vi "Milling parameter to trapezoidal shape.vi"(6 "Y location (um)":dbl, 8 "Image height":u32=512, 9 "Image width":u32=512, 11 "Milling para":T1={"X resolution"=4096, "Y resolution"=125001, "X offset (um)"=0.0, "Y offset (um)"=0.0, "X center (um)"=0.0, "Y center (um)"=0.0, "X size (um)"=250.0, "Y size (um)"=250.0, "UL-Ang"=90.0, "UR-Ang"=90.0, "Line milling time (s)"=5.0, "Z-step (nm)"=2.0, "Lines auto pause"=1, "Auto pause"=FALSE, "Mill from Bottom"=FALSE, "FIB FOV (um)"=500.0, "Auto Profile"=FALSE, "Mill start from Last"=FALSE, "FIB PID on"=FALSE, "FIB PID reset"=TRUE, "FIB PID measured"=0, "FIB PID target"=0.0, "FIB PID target slope"=0.0, "FIB PID P"=0.001, "FIB PID I"=0.01, "FIB PID D"=0.0, "Emission (uA)"=1.36, "Suppressor (V)"=50.0, "Auto reheat"=FALSE} caption="Milling Parameters" {"Suppressor (V)" step=0.1 format="%.1g"; "Emission (uA)" step=0.1 format="%.2g"; "FIB PID measured" items=["Spec.", "B.D. 1", "B.D. 2", "Mill", "Spec. +"]; "FIB PID target slope" min=-1 max=1 step=0.1; "UR-Ang" format="%.2f"; "UL-Ang" format="%.2f"; "Y offset (um)" step=0.02 format="%.3g"; "X offset (um)" step=1 format="%.3g"; "FIB FOV (um)" format="%.3g"; "Line milling time (s)" format="%.1f"; "Y center (um)" format="%#.3g"; "X center (um)" format="%#.3g"}) -> (0 "X end":dbl, 1 "X start":dbl, 2 "X size (um) @ Y":dbl, 3 "Trapezoidal":cluster{"X":i16, "Y":i16}[](array[cluster]), 4 "Total progress":dbl)   [LabVIEW 2018]
panel:
  # "Direction"
  # "Start\nfrom"
  # "<"
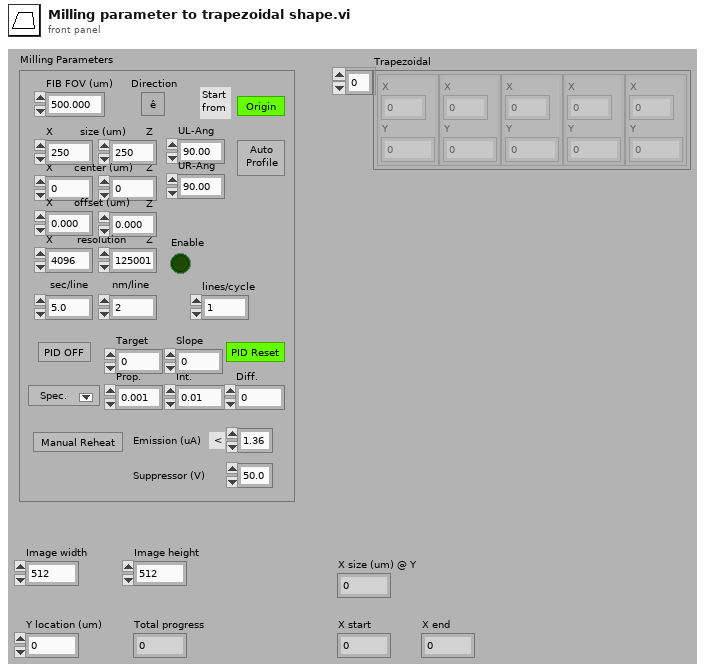
[diagram p1: front panel]
types:
  T1 = cluster{"X resolution":u32, "Y resolution":u32, "X offset (um)":sgl, "Y offset (um)":sgl, "X center (um)":sgl, "Y center (um)":sgl, "X size (um)":sgl, "Y size (um)":sgl, "UL-Ang":sgl, "UR-Ang":sgl, "Line milling time (s)":sgl, "Z-step (nm)":dbl, "Lines auto pause":u16, "Auto pause":bool, "Mill from Bottom":bool, "FIB FOV (um)":sgl, "Auto Profile":bool, "Mill start from Last":bool, "FIB PID on":bool, "FIB PID reset":bool, "FIB PID measured":u8, "FIB PID target":sgl, "FIB PID target slope":sgl, "FIB PID P":sgl, "FIB PID I":sgl, "FIB PID D":sgl, "Emission (uA)":dbl, "Suppressor (V)":sgl, "Auto reheat":bool}
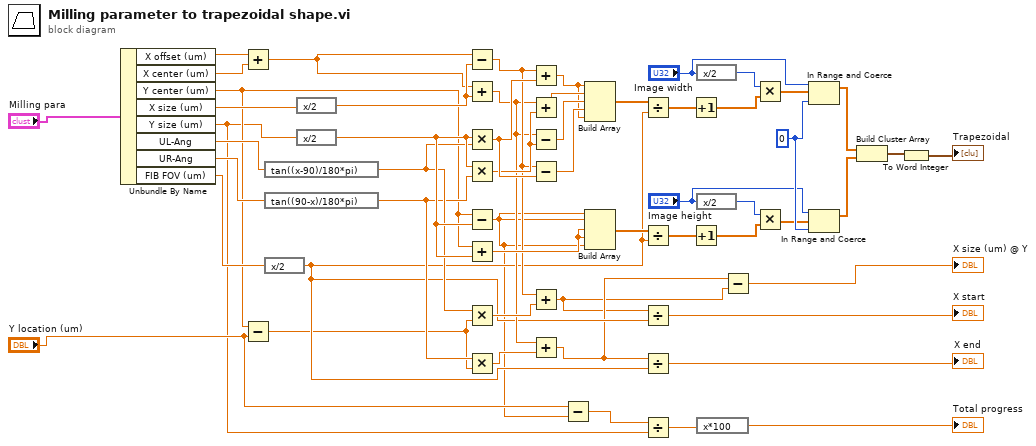
[diagram p0: block diagram]
diagram:
  w33 = u32 0 ("Image width")
  n1 = Unbundle By Name("Milling para") -> ("X offset (um)"=w10:sgl, "X center (um)"=w9:sgl, "Y center (um)"=w11:sgl, "X size (um)"=w54:sgl, "Y size (um)"=w4:sgl, "UL-Ang"=w53:sgl, "UR-Ang"=w52:sgl, "FIB FOV (um)"=w25:sgl)
  n2 = Add(x=w10, y=w9) -> (x+y=w8:sgl)
  n3 = Subtract(x=w11, y="Y location (um)") -> (x-y=w12:dbl)
  n4 = expression code="tan((x-90)/180*pi)"(w53) -> (w24:sgl)
  n5 = expression code="tan((90-x)/180*pi)"(w52) -> (w23:sgl)
  n6 = expression code="x/2"(w25) -> (w17:sgl)
  n7 = expression code="x/2"(w54) -> (w51:sgl)
  n8 = expression code="x/2"(w4) -> (w44:sgl)
  n9 = Subtract(x=w8, y=w51) -> (x-y=w22:sgl)
  n10 = Add(x=w8, y=w51) -> (x+y=w20:sgl)
  n11 = Multiply(x=w44, y=w24) -> (x*y=w50:sgl)
  n12 = Multiply(x=w44, y=w23) -> (x*y=w49:sgl)
  n13 = Subtract(x=w11, y=w44) -> (x-y=w6:sgl)
  n14 = Add(x=w11, y=w44) -> (x+y=w43:sgl)
  n15 = Multiply(x=w24, y=w12) -> (x*y=w21:dbl)
  n16 = Multiply(x=w23, y=w12) -> (x*y=w19:dbl)
  n17 = Add(x=w22, y=w50) -> (x+y=w45:sgl)
  n18 = Add(x=w20, y=w49) -> (x+y=w48:sgl)
  n19 = Subtract(x=w20, y=w49) -> (x-y=w47:sgl)
  n20 = Subtract(x=w22, y=w50) -> (x-y=w46:sgl)
  n21 = Add(x=w22, y=w21) -> (x+y=w14:dbl)
  n22 = Add(x=w20, y=w19) -> (x+y=w15:dbl)
  n23 = Subtract(x="Y location (um)", y=w6) -> (x-y=w5:dbl)
  n24 = Build Array(w45, w48, w47, w46, w45) -> (w42:sgl[])
  n25 = Build Array(w6, w6, w43, w43, w6) -> (w38:sgl[])
  n26 = Divide(x=w42, y=w17) -> (x/y=w41:sgl[])
  n27 = Divide(x=w38, y=w17) -> (x/y=w39:sgl[])
  n28 = Divide(x=w14, y=w17) -> (x/y=→"X start":dbl)
  n29 = Divide(x=w15, y=w17) -> (x/y=→"X end":dbl)
  n30 = Divide(x=w5, y=w4) -> (x/y=w3:dbl)
  n31 = Increment(x=w41) -> (x+1=w40:sgl[])
  n32 = Increment(x=w39) -> (x+1=w37:sgl[])
  n33 = expression code="x/2"("Image width") -> (w36:u32)
  n34 = expression code="x/2"("Image height") -> (w34:u32)
  n35 = expression code="x*100"(w3) -> (→"Total progress":dbl)
  n36 = Subtract(x=w15, y=w14) -> (x-y=→"X size (um) @ Y":dbl)
  n37 = Multiply(x=w36, y=w40) -> (x*y=w31:sgl[])
  n38 = Multiply(x=w34, y=w37) -> (x*y=w30:sgl[])
  n39 = In Range and Coerce(upper limit="Image width", x=w31, lower limit=w33) -> (coerced(x)=w35:sgl[])  [unwired: 1 out]
  n40 = In Range and Coerce(upper limit="Image height", x=w30, lower limit=w33) -> (coerced(x)=w32:sgl[])  [unwired: 1 out]
  n41 = Build Cluster Array(w35, w32) -> (w29:cluster{"Image width":sgl, "Image width":sgl}[])
  n42 = To Word Integer(number=w29) -> (16bit integer=→"Trapezoidal":cluster{"Image width":i16, "Image width":i16}[])
